vi "tearDown.vi"(8 "error in (no error)":errorcluster, 11 "LUnit test In":refnum<class "LUnit Test 4.lvclass">) -> (0 "error out":errorcluster, 3 "LUnit test Out":refnum<class "LUnit Test 4.lvclass">)   [LabVIEW 2020, in "LUnit Test 4.lvclass"]
uses:
  LUnit Test 4.lvclass
  <vilib>/Astemes/LUnit/Test Case.lvclass
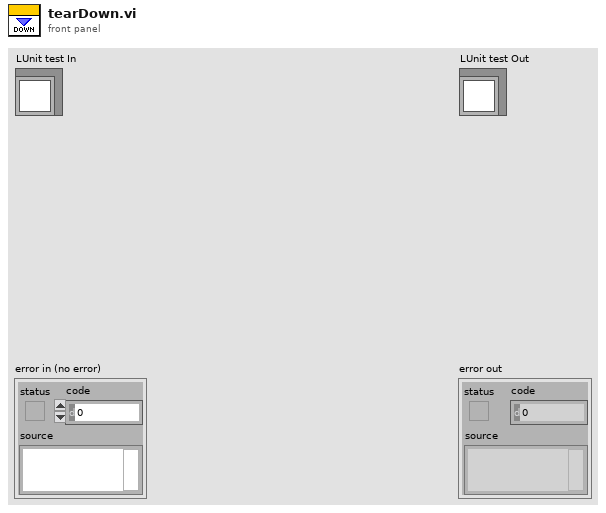
[diagram p1: front panel]
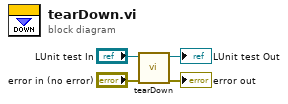
[diagram p0: block diagram]
diagram:
  n1 = call-parent "tearDown.vi"("error in (no error)"="error in (no error)", "LUnit Test Case In"="LUnit test In") -> ("error out"=→"error out":errorcluster, "LUnit Test Case Out"=→"LUnit test Out":refnum<class "LUnit Test 4.lvclass">)  [unwired: 8 in]
